vi "UHR-Fleezers Control (host) - 12.6.vi"() -> ()   [LabVIEW 2012] (continued)
                n2798 = xnode "Read/Write Control"("FPGA VI Reference In"=w3561, "error in"=w3560, "FPGA Trap Trig"=w3557) -> ("FPGA VI Reference Out"=w3559:T20, "error out"=w3558:errorcluster)
                n2799 = xnode "Read/Write Control"("FPGA VI Reference In"=w3559, "error in"=w3558, "TTrig?"=w3557) -> ()  [unwired: 2 out]
              }
            }
            n2800 = Select(t="Wait for trigger", s=w3544, f="Initialize") -> (s? t:f=w3552:string)
            n2801 = case shown="True" w3544 {
              tunnel: w3545 -> [_ w3564]
              tunnel: w3543 -> [_ w3573]
              tunnel: w3542 -> [_ w3572]
              frame False {
                n2802 = local write "Waiting"(FALSE ("Waiting")) -> ()
                "Initializing" <- TRUE ("Initializing")
              }
              frame True {
                n2803 = local read "Threshold (nm)"() -> (w3576:dbl)
                n2804 = local read "AOM X Cal (nm/MHz)"() -> (w3575:dbl)
                n2805 = Add(x=w3564, y=w3576) -> (x+y=w3577:dbl)
                n2806 = Divide(x=w3577, y=w3575) -> (x/y=w3574:dbl)
                n2807 = call "IR AOM freq to word.vi"("Frequency In (MHz)"=w3574) -> ("Frequency Word Out (double)"=w3571:dbl)
                n2808 = local write "Initializing"(FALSE ("Initializing")) -> ()
                n2809 = local write "Waiting"(TRUE ("Waiting")) -> ()
                n2810 = To Quad Integer(1:w3571) -> (0:w3570:i64)
                n2811 = xnode "Read/Write Control"("FPGA VI Reference In"=w3573, "error in"=w3572, "FPGA TTrig Thresh"=w3570) -> ("FPGA VI Reference Out"=w3567:T20, "error out"=w3566:errorcluster)
                n2812 = xnode "Read/Write Control"("FPGA VI Reference In"=w3567, "error in"=w3566, "FPGA Trap Trig"=TRUE) -> ()  [unwired: 2 out]
              }
            }
          }
        }
      }
    }
    n2813 = feedback-in #23(w3153) -> ()
    n2814 = feedback-in #24(w3150) -> ()
    n2815 = Split 1D Array(array=w3105, index=w3167) -> (first subarray=w3268:dbl[])  [unwired: 1 out]
    n2816 = feedback-in #25(w3268) -> ()
    n2817 = call-poly <vilib>:"Mean.vi"("X"=w3268) -> ("mean"=w3267:dbl)  [unwired: 1 out]
    "Bead Mean (nm)" <- w3267
    n2818 = Subtract(x=w3268, y=w3267) -> (x-y=w3266:dbl[])
    n2819 = Square(x=w3266) -> (x^2=w3265:dbl[])
    n2820 = call-poly <vilib>:"Mean.vi"("X"=w3265) -> ("mean"=w3264:dbl)  [unwired: 1 out]
    n2821 = Square Root(x=w3264) -> (sqrt(x)=w3263:dbl)
    n2822 = Multiply(x=10.0, y=w3263) -> (x*y=→"RMS (Ang)":dbl)
    n2823 = xnode ("Read/Write Control")("FPGA VI Reference In"=w3300, "error in"=w3299) -> ("FPGA VI Reference Out"=w3135:T20, "error out"=w3134:errorcluster, "AI2 Y Sum Set 1"=w3398:i16, "AI2 Y Sum Set 2"=w3397:i16, "AI1 X Set 1"=w3199:fxp<+/-,16,1>, "AI1 X Set 2"=w3198:fxp<+/-,16,1>, "Trap Pos FB Int Signal"=→"Trap Pos FB Int Signal":fxp<+/-,24,9>, "Trap Pos FB Int-Norm Signal"=→"Trap Pos FB Int-Norm Signal":fxp<+/-,16,1>, "Trap Pos FB Action"=w3192:i64, "Scanning"=→"AOD Scanning":bool, "Scan I"=→"AOD Scan I":u64, "Scanning MCL"=w3400:bool, "Scan I (MCL)"=→"MCL Scan I":u64, "Green FB Sum"=w3337:i16, "Trap Pos FB Action"=w3122:i64, "TTrig Fin Thresh"=w3118:i64, "Red FB Intensity"=w3099:i16, "Blue Intensity"=w3094:i16)
    "MCL Scanning" <- w3400
    "Trap Pos FB Action" <- w3192
    n2824 = Divide(x=w3099, y=3276.7) -> (x/y=w3098:dbl)
    "Red laser intensity (V)" <- w3098
    n2825 = Divide(x=w3094, y=3276.7) -> (x/y=w3093:dbl)
    "Blue laser intensity (V)" <- w3093
    n2826 = Divide(x=w3337, y=3276.7) -> (x/y=w3097:dbl)
    "Green laser intensity (V)" <- w3097
    n2827 = local read "FB Trig Integrate"() -> (w3116:u32)
    n2828 = Divide(x=w3122, y=w3116) -> (x/y=w3115:dbl)
    "TTrig Sig (Int)" <- w3115
    n2829 = Bundle(w3097, w3098, w3093) -> (→"Fluorescence laser intensities plot":cluster{dbl, dbl, dbl})  [unwired: 1 in]
    n2830 = Divide(x=w3118, y=w3116) -> (x/y=w3113:dbl)
    "TTrig Fin Thresh (Int)" <- w3113
    n2831 = local read "AOM X Cal (nm/MHz)"() -> (w3121:dbl)
    n2832 = local read "AI2 (V)"() -> (w3399:cluster{"Set 1":dbl, "Set 2":dbl})
    n2833 = Bundle By Name(cluster=w3399, "Set 1"=w3398, "Set 2"=w3397) -> (w3395:cluster{"Set 1":dbl, "Set 2":dbl})
    n2834 = Divide(x=w3192, y=327.67) -> (x/y=→"Action (%)":dbl)
    n2835 = local read "Trap X (AI1)"() -> (w3212:T10)
    n2836 = call "IR AOM word double to freq.vi"("Frequency Word In (double)"=w3113) -> ("Frequency Out (MHz)"=w3112:dbl)
    n2837 = call "IR AOM word double to freq.vi"("Frequency Word In (double)"=w3115) -> ("Frequency Out (MHz)"=w3114:dbl)
    n2838 = Divide(x=w3395, y=3276.7) -> (x/y=w3394:cluster{"Set 1":dbl, "Set 2":dbl})
    n2839 = Multiply(x=w3114, y=w3121) -> (x*y=w3120:dbl)
    "TTrig Sig (nm)" <- w3120
    n2840 = Multiply(x=w3112, y=w3121) -> (x*y=w3119:dbl)
    "TTrig Fin Thresh (nm)" <- w3119
    n2841 = local write "AI2 (V)"(w3394) -> ()
    n2842 = Bundle(cluster=w3212, "Trap 1"=w3199, "Trap 2"=w3198) -> (→"Trap X (AI1)":T10)
    n2843 = Bundle(w3120, w3119) -> (→"TTrig":cluster{dbl, dbl})  [unwired: 1 in]
    n2844 = flat-sequence "To save data" {
      tunnel: [w4484] -> w3418
      tunnel: [w4485] -> w3417
      tunnel: w3368 -> [w4478]
      tunnel: w3140 -> [w4482]
      tunnel: ["Save Calibration"] -> w3391
      tunnel: w3388 -> [w4481]
      tunnel: [w4474] -> w3387
      tunnel: [w4471] -> w3386
      tunnel: [w4468] -> w3385
      tunnel: w3367 -> [w4470]
      tunnel: w3282 -> [w4464]
      tunnel: [w4464] -> w3281
      tunnel: ["Start Saving"] -> w3251
      tunnel: [w4458] -> w3180
      tunnel: [w4457] -> w3179
      tunnel: w3418 -> [w4732]
      tunnel: w3417 -> [w4731]
      tunnel: w3181 -> [w4730]
      tunnel: w3391 -> [w4729]
      tunnel: w3387 -> [w4727]
      tunnel: w3386 -> [w4726]
      tunnel: w3385 -> [w4725]
      tunnel: w3260 -> [w4724]
      tunnel: w3292 -> [w4723]
      tunnel: w3281 -> [w4722]
      tunnel: w3251 -> [w4721]
      tunnel: w3249 -> [w4720]
      tunnel: w3077 -> [w4719]
      tunnel: w3180 -> [w4718]
      tunnel: w3179 -> [w4717]
      tunnel: w3178 -> [w4716]
      tunnel: w3101 -> [w4715]
      frame #0 {
        n2845 = Or(x="Save N Sets", y="Start Saving") -> (x .or. y?=w4465:bool)
        n2846 = To Double Precision Float(number=w4481) -> (double precision float=w4475:dbl)
        n2847 = Build Array(w4465, "Save Calibration", w4478, w4470) -> (w4480:bool[])
        n2848 = Compound Arithmetic op=OR("Save Calibration", w4478, w4465, w4470) -> (w4483:bool)
        n2849 = Boolean Array To Number(Boolean array=w4480) -> (number=w4477:u32)
        n2850 = feedback #27(FALSE ("Save APD Data\nwith Trap Data")) -> (w4459:bool)
        n2851 = feedback #28(refnum<k0> refnum) -> (w4486:refnum<file>)
        n2852 = feedback #29(refnum<k0> refnum) -> (w4461:refnum<file>)
        n2853 = feedback #30(FALSE ("Save APD Data\nwith Trap Data")) -> (w4469:bool)
        n2854 = feedback #31(refnum<k0> refnum) -> (w4472:refnum<file>)
        n2855 = feedback #32(0) -> (w4488:i32)
        n2856 = feedback #33() -> (w4476:u32)  [unwired: 1 out]
        n2857 = case shown="True" w4483 {
          tunnel: [w4495 1] -> w4484
          tunnel: w4488 -> [w4497 _]
          tunnel: [w4496 w4528] -> w4485
          tunnel: w4486 -> [w4496 _]
          tunnel: w4482 -> [_ w4546]
          tunnel: w4475 -> [_ w4544]
          tunnel: w4477 -> [_ w4547]
          tunnel: [w4494 w4527] -> w4474
          tunnel: w4476 -> [w4494 _]
          tunnel: [w4493 w4525] -> w4471
          tunnel: w4472 -> [w4493 _]
          tunnel: [w4492 w4524] -> w4468
          tunnel: w4469 -> [w4492 _]
          tunnel: "Start Saving" -> [_ w4522]
          tunnel: w4464 -> [_ w4521]
          tunnel: [w4491 w4513] -> w4457
          tunnel: w4461 -> [w4491 _]
          tunnel: [w4490 w4512] -> w4458
          tunnel: w4459 -> [w4490 _]
          frame False {
            n2858 = Increment(x=w4497) -> (x+1=w4495:i32)
          }
          frame True {
            w4518 = FALSE ("Start Saving")
            w4523 = 9.0  # File Version
            w4530 = FALSE ("prepend array or string size? (T)")
            w4529 = T28."big-endian, network order" ("byte order (0:big-endian, network order)")
            n2859 = local read "BD 1 Frequency 1 (MHz)"() -> (w4543:dbl)
            n2860 = local read "BD 2 Frequency 1 (MHz)"() -> (w4542:dbl)
            n2861 = local read "BD 1 Frequency 2 (MHz)"() -> (w4541:dbl)
            n2862 = local read "BD 2 Frequency 2 (MHz)"() -> (w4540:dbl)
            n2863 = local read "BD 1 Frequency 3 (MHz)"() -> (w4539:dbl)
            n2864 = local read "BD 2 Frequency 3 (MHz)"() -> (w4538:dbl)
            n2865 = Array Size(array=w4521) -> (size(s)=w4520:i32)
            n2866 = To Double Precision Float(number=w4520) -> (double precision float=w4519:dbl)
            n2867 = local write "Save Calibration"(w4518) -> ()
            n2868 = local write "Start Saving"(w4518) -> ()
            n2869 = Build Array("Save APD Data\nwith Trap Data", "Save Trap Pos. Data") -> (w4515:bool[])
            n2870 = Boolean Array To Number(Boolean array=w4515) -> (number=w4514:u32)
            n2871 = Build Array(w4543, w4542, w4541, w4540, w4539, w4538) -> (w4537:dbl[])
            n2872 = case shown="1, Default" w4547 {
              tunnel: w4546 -> [w4619 w4639 w4655 w4693]
              tunnel: w4519 -> [w4624 w4646 w4675 w4712]
              tunnel: w4544 -> [w4623 w4645 w4674 w4711]
              tunnel: [w4620 w4641 w4666 w4703] -> w4535
              tunnel: [w4611 "Cal sets to save" w4656 w4694] -> w4527
              tunnel: w4537 -> [w4621 w4642 w4668 w4705]
              tunnel: "Save APD Data\nwith Trap Data" -> [w4618 _ w4652 w4691]
              tunnel: [w4618 w4633 w4652 w4691] -> w4524
              tunnel: w4523 -> [w4614 w4634 w4650 w4689]
              tunnel: w4522 -> [w4613 _ _ _]
              tunnel: [w4604 w4633 w4649 w4679] -> w4512
              tunnel: "Save Trap Pos. Data" -> [w4604 _ w4649 w4679]
              tunnel: w4514 -> [w4603 _ w4648 w4678]
              frame 1, Default {
                # "timeseries"
                n2873 = case shown="True" "Profile" {
                  tunnel: [w4627 w4631] -> w4608
                  tunnel: [w4627 w4630] -> w4607
                  tunnel: [w4627 w4629] -> w4606
                  tunnel: [w4627 w4628] -> w4605
                  frame False {
                    w4627 = 0.0 ("f")
                  }
                  frame True {
                    n2874 = local read "Current Position"() -> (w4632:cluster{dbl, dbl, dbl})
                    n2875 = local read "Y change (mm)"() -> (w4628:dbl)
                    n2876 = Unbundle(w4632) -> (w4631:dbl, w4630:dbl, w4629:dbl)
                  }
                }
                n2877 = local read "Save ave N"() -> (w4626:dbl)
                n2878 = Multiply(x=w4626, y=w4619) -> (x*y=w4625:dbl)
                n2879 = To Double Precision Float(number=w4603) -> (double precision float=w4617:dbl)
                n2880 = Build Array(w4614, w4619, w4625, w4624, w4623, 0.0 ("f")) -> (w4622:dbl[])
                n2881 = Build Array(w4617, w4608, w4607, w4606, w4605) -> (w4615:dbl[])
                n2882 = Select(t=u32 4000000000, s=w4613, f="N sets to save") -> (s? t:f=w4611:u32)
                n2883 = Build Array (concatenate)(w4622, w4621, w4615) -> (w4620:dbl[])
              }
              frame 2 {
                w4636 = 0.0 ("f")
                w4633 = FALSE ("Save APD Data\nwith Trap Data")
                # "calibration"
                n2884 = Boolean To (0,1)(Boolean=w4633) -> (0, 1=w4638:i16)
                n2885 = To Double Precision Float(number=w4638) -> (double precision float=w4637:dbl)
                n2886 = Build Array(w4637, w4636, w4636, w4636, w4636) -> (w4635:dbl[])
                n2887 = Build Array(w4634, w4639, w4639, w4646, w4645, 1.0 ("t")) -> (w4643:dbl[])
                n2888 = Build Array (concatenate)(w4643, w4642, w4635) -> (w4641:dbl[])
                "Calibrating Trap..." <- TRUE ("Calibrating...")
              }
              frame 4 {
                w4653 = 0.0 ("f")
                # "scan dir (x/y = 0/1)"
                # "cycles/step"
                # "n scans (f/b)"
                # "steps"
                # "freq. range"
                # "AOD raster scan"
                n2889 = local read "Number of F/B Scans (AOD)"() -> (w4660:u16)
                n2890 = local read "Cycles/step (AOD)"() -> (w4662:u64)
                n2891 = local read "Scan Range (MHz)"() -> (w4665:dbl)
                n2892 = local read "Scan steps (AOD)"() -> (w4664:u64)
                n2893 = local read "Scan BD"() -> (w4672:bool)
                n2894 = local read "Save ave N"() -> (w4677:dbl)
                n2895 = Boolean To (0,1)(Boolean=w4672) -> (0, 1=w4671:i16)
                n2896 = To Double Precision Float(number=w4660) -> (double precision float=w4659:dbl)
                n2897 = To Double Precision Float(number=w4664) -> (double precision float=w4663:dbl)
                n2898 = To Double Precision Float(number=w4662) -> (double precision float=w4661:dbl)
                n2899 = To Double Precision Float(number=w4671) -> (double precision float=w4670:dbl)
                n2900 = Multiply(x=w4677, y=w4655) -> (x*y=w4676:dbl)
                n2901 = To Double Precision Float(number=w4648) -> (double precision float=w4654:dbl)
                n2902 = Build Array(w4654, w4653, w4653, w4653, w4653) -> (w4651:dbl[])
                n2903 = local read "N sets should be saved"() -> (w4657:dbl)
                n2904 = Build Array(w4670, w4665, w4663, w4661, w4659) -> (w4667:dbl[])
                n2905 = Build Array(w4650, w4655, w4676, w4675, w4674, 2.0 ("t")) -> (w4669:dbl[])
                n2906 = Round Toward +Infinity(x=w4657) -> (ceil(x): smallest int >= x=w4658:dbl)
                n2907 = Build Array (concatenate)(w4669, w4668, w4651, w4667) -> (w4666:dbl[])
                n2908 = To Unsigned Long Integer(number=w4658) -> (unsigned 32bit integer=w4656:u32)
              }
              frame 8 {
                w4686 = 0.0 ("f")
                # "MCL raster scan"
                n2909 = local read "Number of scans (MCL)"() -> (w4681:u64)
                n2910 = local read "Scan lines (y)"() -> (w4680:u64)
                n2911 = local read "2D or 1D Scan"() -> (w4683:bool)
                n2912 = local read "Scan Range (V)\n(of steps)"() -> (w4702:dbl)
                n2913 = local read "Fast Scan Dir"() -> (w4709:bool)
                n2914 = local read "Cycles/step (MCL)"() -> (w4699:u64)
                n2915 = local read "Scan steps (MCL)"() -> (w4701:u64)
                n2916 = Select(t=w4680, s=w4683, f=w4681) -> (s? t:f=w4682:u64)
                n2917 = Boolean To (0,1)(Boolean=w4683) -> (0, 1=w4685:i16)
                n2918 = local read "Save ave N"() -> (w4714:dbl)
                n2919 = local read "Initial X"() -> (w4688:dbl)
                n2920 = local read "Initial Y"() -> (w4687:dbl)
                n2921 = To Double Precision Float(number=w4685) -> (double precision float=w4684:dbl)
                n2922 = Boolean To (0,1)(Boolean=w4709) -> (0, 1=w4708:i16)
                n2923 = To Double Precision Float(number=w4682) -> (double precision float=w4697:dbl)
                n2924 = To Double Precision Float(number=w4701) -> (double precision float=w4700:dbl)
                n2925 = To Double Precision Float(number=w4699) -> (double precision float=w4698:dbl)
                n2926 = To Double Precision Float(number=w4708) -> (double precision float=w4707:dbl)
                n2927 = Multiply(x=w4714, y=w4693) -> (x*y=w4713:dbl)
                n2928 = To Double Precision Float(number=w4678) -> (double precision float=w4692:dbl)
                n2929 = local read "N sets should be saved (MCL)"() -> (w4695:dbl)
                n2930 = Build Array(w4692, w4684, w4686, w4686, w4686) -> (w4690:dbl[])
                n2931 = Build Array(w4707, w4702, w4700, w4698, w4697, w4688, w4687) -> (w4704:dbl[])
                n2932 = Build Array(w4689, w4693, w4713, w4712, w4711, 3.0 ("t")) -> (w4706:dbl[])
                n2933 = Round Toward +Infinity(x=w4695) -> (ceil(x): smallest int >= x=w4696:dbl)
                n2934 = Build Array (concatenate)(w4706, w4705, w4690, w4704) -> (w4703:dbl[])
                n2935 = To Unsigned Long Integer(number=w4696) -> (unsigned 32bit integer=w4694:u32)
              }
            }
            n2936 = local read "Index"() -> (w4552:dbl)
            n2937 = call "Create new save file.vi"("Insert"="", "Ext"=".dat", "Index In"=w4552) -> ("Path Out"=w4508:path, "Index Out"=w4526:dbl)
            n2938 = local write "Save file name"(w4508) -> ()
            n2939 = local write "Index"(w4526) -> ()
            n2940 = local write "Save index"(w4526) -> ()
            n2941 = Array Size(array=w4535) -> (size(s)=w4536:i32)
            n2942 = Open/Create/Replace File(file path (use dialog)=w4508, operation (0:open)=T29."create", access (0:read/write)=enum16{"read/write", "read-only", "write-only"}."write-only") -> (refnum out=w4549:refnum<file>)  [unwired: 1 in, 4 out]
            n2943 = local write "Saving..."(TRUE ("Saving...")) -> ()
            n2944 = To Double Precision Float(number=w4536) -> (double precision float=w4534:dbl)
            n2945 = String Length(string="Comment (data description)") -> (length=w4533:i32)
            n2946 = To Double Precision Float(number=w4533) -> (double precision float=w4532:dbl)
            n2947 = Deny Access(7:w4549) -> (3:w4548:refnum<file>)  [unwired: 1 in, 2 out]
            n2948 = Build Array (concatenate)(w4534, w4535, w4532) -> (w4507:dbl[])
            n2949 = case "If fluorescence data to be saved" shown="True" w4524 {
              tunnel: w4508 -> [_ w4602]
              tunnel: [refnum<k0> refnum w4582] -> w4525
              frame False {
              }
              frame True {
                w4581 = 0.0
                n2950 = local read "APD Integration Time (s)"() -> (w4587:dbl)
                n2951 = local read "N APD Samp/step"() -> (w4580:dbl)
                n2952 = local read "Number of APDs"() -> (w4579:u8)
                n2953 = Path To String(path=w4602) -> (string=w4601:string)
                n2954 = String Length(string=w4601) -> (length=w4600:i32)
                n2955 = Subtract(x=w4600, y=4) -> (x-y=w4598:i32)
                n2956 = String Subset(string=w4601, length (rest)=w4598) -> (substring=w4597:string)  [unwired: 1 out]
                n2957 = Build Array(w4587, w4580, w4579, w4581, w4581, w4581, w4581, w4581) -> (w4584:dbl[])
                n2958 = Concatenate Strings(w4597, "_fl.dat" ("string")) -> (w4595:string)
                n2959 = Array Size(array=w4584) -> (size(s)=w4586:i32)
                n2960 = String To Path(string=w4595) -> (path=w4591:path)
                n2961 = Open/Create/Replace File(file path (use dialog)=w4591, operation (0:open)=T29."create", access (0:read/write)=enum16{"read/write", "read-only", "write-only"}."write-only") -> (refnum out=w4592:refnum<file>)  [unwired: 1 in, 4 out]
                n2962 = Deny Access(7:w4592) -> (3:w4588:refnum<file>)  [unwired: 1 in, 2 out]
                n2963 = To Double Precision Float(number=w4586) -> (double precision float=w4585:dbl)
                n2964 = Build Array (concatenate)(w4585, w4584) -> (w4583:dbl[])
                n2965 = Write to Binary File(file (use dialog)=w4588, data=w4583, 5:FALSE ("prepend array or string size? (T)"), 9:T28."big-endian, network order" ("byte order (0:big-endian, network order)")) -> (refnum out=w4582:refnum<file>)  [unwired: 1 in, 3 out]
              }
            }
            n2966 = case shown="True" w4512 {
              tunnel: w4508 -> [_ w4563]
              tunnel: [refnum<k0> refnum w4562] -> w4513
              frame False {
              }
              frame True {
                w4558 = 0.0 ("element")
                n2967 = Path To String(path=w4563) -> (string=w4577:string)
                n2968 = Build Array(w4558, w4558, w4558, w4558, w4558, w4558, w4558, w4558) -> (w4559:dbl[])
                n2969 = String Length(string=w4577) -> (length=w4576:i32)
                n2970 = Subtract(x=w4576, y=4) -> (x-y=w4574:i32)
                n2971 = Array Size(array=w4559) -> (size(s)=w4561:i32)
                n2972 = String Subset(string=w4577, length (rest)=w4574) -> (substring=w4573:string)  [unwired: 1 out]
                n2973 = To Double Precision Float(number=w4561) -> (double precision float=w4560:dbl)
                n2974 = Concatenate Strings(w4573, "_pos.dat" ("string")) -> (w4571:string)
                n2975 = Build Array (concatenate)(w4560, w4559) -> (w4557:dbl[])
                n2976 = String To Path(string=w4571) -> (path=w4567:path)
                n2977 = Open/Create/Replace File(file path (use dialog)=w4567, operation (0:open)=T29."create", access (0:read/write)=enum16{"read/write", "read-only", "write-only"}."write-only") -> (refnum out=w4568:refnum<file>)  [unwired: 1 in, 4 out]
                n2978 = Deny Access(7:w4568) -> (3:w4564:refnum<file>)  [unwired: 1 in, 2 out]
                n2979 = Write to Binary File(file (use dialog)=w4564, data=w4557, 5:FALSE ("prepend array or string size? (T)"), 9:T28."big-endian, network order" ("byte order (0:big-endian, network order)")) -> (refnum out=w4562:refnum<file>)  [unwired: 1 in, 3 out]
              }
            }
            n2980 = Write to Binary File(file (use dialog)=w4548, data=w4507, 5:w4530, 9:w4529) -> (refnum out=w4531:refnum<file>)  [unwired: 1 in, 3 out]
            n2981 = Write to Binary File(file (use dialog)=w4531, data="Comment (data description)", 5:w4530, 9:w4529) -> (refnum out=w4528:refnum<file>)  [unwired: 1 in, 3 out]
            n2982 = local read "connection reference"() -> (w4510:T17)
            n2983 = Bundle("Comment (data description)"="Comment (data description)", "Channel 1 Buffer"="Channel 1 Buffer", "Channel 2 Buffer"="Channel 2 Buffer", "Channel 3 Buffer"="Channel 3 Buffer", "Title"="Title", "DNA Construct"="DNA Construct", "Bead diameter"="Bead diameter", "Name"="Name") -> (w4498:T47)  [unwired: 1 in]
            n2984 = call "MattFileCreator-v9.vi"("Comments"=w4498, "Input Array"=w4507, "File path"=w4508, "table"="labview", "connection reference"=w4510) -> ("connection reference out"=w4509:T17)  [unwired: 5 in, 1 out]
            n2985 = local write "connection reference"(w4509) -> ()
          }
        }
        n2986 = feedback-in #27(w4458) -> ()
        n2987 = feedback-in #28(w4485) -> ()
        n2988 = feedback-in #29(w4457) -> ()
        n2989 = feedback-in #30(w4468) -> ()
        n2990 = feedback-in #31(w4471) -> ()
        n2991 = feedback-in #32(w4484) -> ()
        n2992 = feedback-in #33(w4474) -> ()
      }
      frame #1 {
        n2993 = local read "Saving..."() -> (w4728:bool)
        n2994 = case shown="True" w4728 {
          tunnel: w4732 -> [_ w4743]
          tunnel: w4731 -> [_ w4757]
          tunnel: w4730 -> [_ w4753]
          tunnel: w4729 -> [_ w4752]
          tunnel: w4727 -> [_ w4751]
          tunnel: w4726 -> [_ w4746]
          tunnel: w4725 -> [_ w4745]
          tunnel: w4724 -> [_ w4744]
          tunnel: w4723 -> [_ w4742]
          tunnel: w4722 -> [_ w4740]
          tunnel: w4721 -> [_ w4739]
          tunnel: w4720 -> [_ w4738]
          tunnel: w4719 -> [_ w4737]
          tunnel: w4718 -> [_ w4736]
          tunnel: w4717 -> [_ w4735]
          tunnel: w4716 -> [_ w4734]
          tunnel: w4715 -> [_ w4733]
          frame False {
          }
          frame True {
            n2995 = Multiply(x=w4743, y=w4742) -> (x*y=→"Time (s)":dbl)
            n2996 = Less Or Equal?(x=w4743, y=w4751) -> (x <= y?=w4755:bool)
            n2997 = Or(x="Stop Saving", y="Abort save 2") -> (x .or. y?=w4747:bool)
            n2998 = Not(x=w4747) -> (.not. x?=w4756:bool)
            n2999 = And(x=w4755, y=w4756) -> (x .and. y?=w4754:bool)
            n3000 = case shown="True" w4754 {
              tunnel: w4757 -> [w4764 w4855]
              tunnel: [0.0 w4858] -> w4750
              tunnel: w4743 -> [_ w4856]
              tunnel: w4751 -> [_ w4857]
              tunnel: w4753 -> [_ w4852]
              tunnel: w4752 -> [_ _]
              tunnel: w4746 -> [w4762 w4845]
              tunnel: w4745 -> [w4761 w4846]
              tunnel: w4744 -> [_ w4844]
              tunnel: w4740 -> [_ w4843]
              tunnel: w4739 -> [_ w4767]
              tunnel: w4738 -> [_ w4836]
              tunnel: w4737 -> [_ w4783]
              tunnel: w4736 -> [w4758 w4800]
              tunnel: w4735 -> [w4759 w4799]
              tunnel: w4734 -> [_ w4796]
              tunnel: w4733 -> [_ w4794]
              frame False {
                w4760 = FALSE
                n3001 = Close File(refnum=w4764) -> ()  [unwired: 1 in, 2 out]
                n3002 = case shown="True" w4761 {
                  tunnel: w4762 -> [_ w4766]
                  frame False {
                  }
                  frame True {
                    n3003 = Close File(refnum=w4766) -> ()  [unwired: 1 in, 2 out]
                  }
                }
                n3004 = case shown="True" w4758 {
                  tunnel: w4759 -> [_ w4765]
                  frame False {
                  }
                  frame True {
                    n3005 = Close File(refnum=w4765) -> ()  [unwired: 1 in, 2 out]
                  }
                }
                n3006 = local write "Raster Scanning..."(w4760) -> ()
                n3007 = local write "Calibrating Trap..."(w4760) -> ()
                n3008 = call <vilib>:"Beep.vi"() -> ()  [unwired: 3 in, 9 out]
                n3009 = local write "Stop Saving"(w4760) -> ()
                "Saving..." <- w4760
              }
              frame True {
                n3010 = local read "Calibrating Trap..."() -> (w4847:bool)
                n3011 = case "Write fl. data" shown="True" w4846 {
                  tunnel: w4845 -> [_ w4881]
                  tunnel: w4844 -> [_ w4880]
                  frame False {
                  }
                  frame True {
                    n3012 = Write to Binary File(file (use dialog)=w4881, data=w4880, 5:FALSE ("prepend array or string size? (T)"), 9:T28."big-endian, network order" ("byte order (0:big-endian, network order)")) -> ()  [unwired: 1 in, 4 out]
                  }
                }
                n3013 = Greater?(x="Save ave N", y=1.0) -> (0:w4850:bool)
                n3014 = Not(x=w4847) -> (.not. x?=w4849:bool)
                n3015 = And(x=w4849, y=w4850) -> (x .and. y?=w4797:bool)
                n3016 = case shown="True" w4797 {
                  tunnel: w4796 -> [w4861 w4872]
                  tunnel: [w4861 w4864] -> w4795
                  tunnel: "Save ave N" -> [_ w4865]
                  frame False {
                  }
                  frame True {
                    w4862 = 2 ("dimension size")
                    n3017 = Array Size(array=w4872) -> (size(s)=w4866:i32)
                    n3018 = Divide(x=w4866, y=w4862) -> (x/y=w4870:dbl)
                    n3019 = Reshape Array(w4872, w4870, w4862) -> (w4871:u64[][])
                    n3020 = Transpose 2D Array(2D array=w4871) -> (transposed array=w4869:u64[][])
                    n3021 = for {
                      tunnel: w4869 -> [w4874] mode=indexing
                      tunnel: [w4873] -> w4863 mode=indexing
                      tunnel: w4865 -> [w4875]
                      workers-P: _ -> [_]
                      n3022 = call "downsample 1D array - U64.vi"("Ave N"=w4875, "Array In"=w4874) -> ("Array Out"=w4873:u64[])  [unwired: 1 in]
                    }
                    n3023 = Transpose 2D Array(2D array=w4863) -> (transposed array=w4868:u64[][])
                    n3024 = Divide(x=w4866, y=w4865) -> (x/y=w4867:dbl)
                    n3025 = Reshape Array(w4868, w4867) -> (w4864:u64[])
                  }
                }
                n3026 = case shown="True" w4797 {
                  tunnel: w4852 -> [w4884 w4896]
                  tunnel: [w4884 w4888] -> w4848
                  tunnel: "Save ave N" -> [_ w4889]
                  tunnel: w4843 -> [_ w4887]
                  frame False {
                  }
                  frame True {
                    n3027 = Array Size(array=w4896) -> (size(s)=w4890:i32)
                    n3028 = Array Size(array=w4887) -> (size(s)=w4886:i32)
                    n3029 = Divide(x=w4890, y=w4886) -> (x/y=w4894:dbl)
                    n3030 = Reshape Array(w4896, w4894, w4886) -> (w4895:i16[][])
                    n3031 = Transpose 2D Array(2D array=w4895) -> (transposed array=w4893:i16[][])
                    n3032 = for {
                      tunnel: w4893 -> [w4899] mode=indexing
                      tunnel: [w4898] -> w4885 mode=indexing
                      tunnel: w4889 -> [w4897]
                      workers-P: _ -> [_]
                      n3033 = call "downsample 1D array - I16.vi"("Ave N"=w4897, "Array In"=w4899) -> ("Array Out"=w4898:i16[])  [unwired: 1 out]
                    }
                    n3034 = Transpose 2D Array(2D array=w4885) -> (transposed array=w4892:i16[][])
                    n3035 = Divide(x=w4890, y=w4889) -> (x/y=w4891:dbl)
                    n3036 = Reshape Array(w4892, w4891) -> (w4888:i16[])
                  }
                }
                n3037 = Index Array(array=w4783, index=2) -> (element=w4784:waveform(dbl))
                n3038 = Index Array(array=w4783, index=1) -> (element=w4817:waveform(dbl))
                n3039 = Index Array(array=w4783, index=0) -> (element=w4819:waveform(dbl))
                n3040 = Unbundle By Name(w4784) -> ("Y"=w4786:dbl[])
                n3041 = Unbundle By Name(w4817) -> ("Y"=w4821:dbl[])
                n3042 = Unbundle By Name(w4819) -> ("Y"=w4829:dbl[])
                n3043 = case "Write trap pos. data" shown="True" w4800 {
                  tunnel: w4799 -> [_ w4877]
                  tunnel: w4795 -> [_ w4876]
                  frame False {
                  }
                  frame True {
                    n3044 = Write to Binary File(file (use dialog)=w4877, data=w4876, 5:FALSE ("prepend array or string size? (T)"), 9:T28."big-endian, network order" ("byte order (0:big-endian, network order)")) -> ()  [unwired: 1 in, 4 out]
                  }
                }
                n3045 = Write to Binary File(file (use dialog)=w4855, data=w4848, 5:FALSE ("prepend array or string size? (T)"), 9:T28."big-endian, network order" ("byte order (0:big-endian, network order)")) -> ()  [unwired: 1 in, 4 out]
                n3046 = feedback #34(w4786) -> (w4787:dbl[])
                n3047 = Build Array (concatenate)(w4787, w4786) -> (w4782:dbl[])
                n3048 = Select(t=w4786, s=w4767, f=w4782) -> (s? t:f=w4772:dbl[])
                n3049 = feedback-in #34(w4772) -> ()
                n3050 = feedback #35(w4821) -> (w4823:dbl[])
                n3051 = Build Array (concatenate)(w4823, w4821) -> (w4822:dbl[])
                n3052 = Select(t=w4821, s=w4767, f=w4822) -> (s? t:f=w4811:dbl[])
                n3053 = feedback-in #35(w4811) -> ()
                n3054 = feedback #36(w4829) -> (w4842:dbl[])
                n3055 = Build Array (concatenate)(w4842, w4829) -> (w4841:dbl[])
                n3056 = Select(t=w4829, s=w4767, f=w4841) -> (s? t:f=w4816:dbl[])
                n3057 = feedback-in #36(w4816) -> ()
                n3058 = Divide(x=w4856, y=w4857) -> (x/y=w4859:dbl)
                n3059 = Multiply(x=w4859, y=100.0) -> (x*y=w4858:dbl)
                n3060 = Build Array(w4816, w4811, w4772) -> (→"Saved APD":dbl[][])
                n3061 = Array Size(array=w4816) -> (size(s)=w4834:i32)
                n3062 = Unbundle By Name(w4836) -> ("Y"=w4840:dbl[])
                n3063 = Subtract(x=w4834, y="N pts to average") -> (x-y=w4769:i32)
                n3064 = Multiply(x="N pts to average", y=u16 2) -> (x*y=w4812:u16)
                n3065 = Subtract(x=w4834, y=w4812) -> (x-y=w4770:i32)
                n3066 = feedback #37(w4840) -> (w4839:dbl[])
                n3067 = Build Array (concatenate)(w4839, w4840) -> (w4838:dbl[])
                n3068 = Select(t=w4840, s=w4767, f=w4838) -> (s? t:f=w4837:dbl[])
                "Trap Delta Graph" <- w4837
                n3069 = feedback-in #37(w4837) -> ()
                n3070 = Array Subset(array=w4816, index=w4769, length="N pts to average") -> (w4833:dbl[])
                n3071 = Array Subset(array=w4816, index=w4770, length="N pts to average") -> (w4832:dbl[])
                n3072 = Array Subset(array=w4811, index=w4769, length="N pts to average") -> (w4814:dbl[])
                n3073 = Array Subset(array=w4811, index=w4770, length="N pts to average") -> (w4813:dbl[])
                n3074 = Array Subset(array=w4772, index=w4769, length="N pts to average") -> (w4781:dbl[])
                n3075 = Array Subset(array=w4772, index=w4770, length="N pts to average") -> (w4780:dbl[])
                n3076 = Index Array(array=w4794, index=0) -> (element=w4792:waveform(dbl))
                n3077 = call-poly <vilib>:"Mean.vi"("X"=w4833) -> ("mean"=w4831:dbl)  [unwired: 1 out]
                n3078 = call-poly <vilib>:"Mean.vi"("X"=w4814) -> ("mean"=w4810:dbl)  [unwired: 1 out]
                n3079 = call-poly <vilib>:"Mean.vi"("X"=w4832) -> ("mean"=w4830:dbl)  [unwired: 1 out]
                n3080 = call-poly <vilib>:"Mean.vi"("X"=w4813) -> ("mean"=w4809:dbl)  [unwired: 1 out]
                n3081 = call-poly <vilib>:"Mean.vi"("X"=w4781) -> ("mean"=w4779:dbl)  [unwired: 1 out]
                n3082 = call-poly <vilib>:"Mean.vi"("X"=w4780) -> ("mean"=w4778:dbl)  [unwired: 1 out]
                n3083 = Unbundle By Name(w4792) -> ("Y"=w4790:dbl[])
                n3084 = Subtract(x=w4810, y=w4809) -> (x-y=w4801:dbl)
                "Delta Fl. 2" <- w4801
                n3085 = Subtract(x=w4779, y=w4778) -> (x-y=w4773:dbl)
                "Delta Fl. 3" <- w4773
                n3086 = Subtract(x=w4831, y=w4830) -> (x-y=w4828:dbl)
                "Delta Fl. 1" <- w4828
                n3087 = feedback #38(w4790) -> (w4789:dbl[])
                n3088 = Build Array (concatenate)(w4789, w4790) -> (w4791:dbl[])
                n3089 = Initialize Array(w4828, 1 ("dimension size")) -> (w4825:dbl[])
                n3090 = Initialize Array(w4801, 1 ("dimension size")) -> (w4806:dbl[])
                n3091 = Initialize Array(w4773, 1 ("dimension size")) -> (w4775:dbl[])
                n3092 = Select(t=w4790, s=w4767, f=w4791) -> (s? t:f=w4788:dbl[])
                "Saved trap pos" <- w4788
                n3093 = feedback-in #38(w4788) -> ()
                n3094 = feedback #39(w4825) -> (w4826:dbl[])
                n3095 = Build Array (concatenate)(w4826, w4825) -> (w4824:dbl[])
                n3096 = feedback #40(w4806) -> (w4807:dbl[])
                n3097 = feedback #41(w4775) -> (w4776:dbl[])
                n3098 = Build Array (concatenate)(w4807, w4806) -> (w4805:dbl[])
                n3099 = Build Array (concatenate)(w4776, w4775) -> (w4774:dbl[])
                n3100 = Select(t=w4825, s=w4767, f=w4824) -> (s? t:f=w4804:dbl[])
                n3101 = feedback-in #39(w4804) -> ()
                n3102 = Select(t=w4806, s=w4767, f=w4805) -> (s? t:f=w4803:dbl[])
                n3103 = feedback-in #40(w4803) -> ()
                n3104 = Select(t=w4775, s=w4767, f=w4774) -> (s? t:f=w4768:dbl[])
                n3105 = feedback-in #41(w4768) -> ()
                n3106 = Build Array(w4804, w4803, w4768) -> (→"Save APD Deriv":dbl[][])
              }
            }
            "Progress" <- w4750
            "Progress 2" <- w4750
          }
        }
      }
    }
    n3107 = local read "wait to reset values"() -> (w3402:bool)
    n3108 = Not(x=w3400) -> (.not. x?=w3403:bool)
    n3109 = And(x=w3403, y=w3402) -> (x .and. y?=w3404:bool)
    n3110 = case "Part of MCL raster scanning: returns to initial positions after scan done" shown="True" w3404 {
      tunnel: w3135 -> [w4278 w4285]
      tunnel: [w4278 w4284] -> w3406
      tunnel: w3134 -> [w4277 w4283]
      tunnel: [w4277 w4282] -> w3401
      frame False {
      }
      frame True {
        w4293 = 10.0 ("y")
        w4292 = 32767.0 ("y")
        # "to return scan values\nafter a synchronous \nAOM scan"
        n3111 = local read "AO2"() -> (w4286:dbl)
        n3112 = local read "AO1"() -> (w4287:dbl)
        n3113 = local write "wait to reset values"(FALSE ("wait to reset values")) -> ()
        n3114 = Multiply(x=w4287, y=w4292) -> (x*y=w4289:dbl)
        n3115 = Multiply(x=w4286, y=w4292) -> (x*y=w4291:dbl)
        n3116 = Divide(x=w4289, y=w4293) -> (x/y=w4288:dbl)
        n3117 = Divide(x=w4291, y=w4293) -> (x/y=w4290:dbl)
        n3118 = To Word Integer(number=w4288) -> (16bit integer=w4294:i16)
        n3119 = To Word Integer(number=w4290) -> (16bit integer=w4295:i16)
        n3120 = local read "Total Counts (ticks)"() -> (w4279:u16)
        n3121 = xnode "Read/Write Control"("FPGA VI Reference In"=w4285, "error in"=w4283, "AO1"=w4294, "AO2"=w4295, "MCL count"=w4279) -> ("FPGA VI Reference Out"=w4284:T20, "error out"=w4282:errorcluster)
        n3122 = local read "Scan Range (V)\n(of steps)"() -> (w4280:dbl)
        n3123 = property on="Scan Range (V)\n(of steps)" class="DigNum (strict)"("Val(Sgnl)"=w4280) -> ()  [unwired: 2 in, 2 out]
      }
    }
    n3124 = node-c288() -> ()  [unwired: 2 out]
  }
  n3125 = flat-sequence "Video" {
    tunnel: [w4909] -> w114
    tunnel: w114 -> [w4949]
    frame #0 {
      n3126 = while {
        stop <- w4901 continue-if-true
        n3127 = call "Close Video Capture.vi"() -> ("error code OUT"=w4903:i32)
        n3128 = Equal?(x=w4903, y=0) -> (x = y?=w4901:bool)
      }
      n3129 = local write "Stop All"(FALSE ("Stop All")) -> ()
    }
    frame #1 {
      n3130 = call "DMR_Init.vi"() -> ()  [unwired: 3 out]
    }
    frame #2 {
      w4904 = "DE245428202"  # MSU fleezers card #
      (unwired) "DE019116701"  # Illinois fleezers card #
      # "Setting the destination format to Mono8 makes sure that the image can be displayed in the intensity plot."
      n3131 = call "DMR_GetDevice.vi"("search string IN"=w4904) -> ("device handle OUT"=w4927:i32)  [unwired: 4 in, 2 out]
      n3132 = call "DMR_OpenDevice.vi"("device handle IN"=w4927) -> ("driver handle OUT"=w4910:i32)  [unwired: 4 out]
      n3133 = call "DMR_FindList.vi"("flags IN"=u32 0 ("flags"), "list name IN"="" ("String"), "list type IN"=T48."camera descriptions", "driver handle IN"=w4910) -> ("list handle OUT"=w4913:i32)  [unwired: 2 out]
      n3134 = call "DMR_FindList.vi"("flags IN"=u32 0 ("flags"), "list name IN"="Base", "list type IN"=T48."setting", "driver handle IN"=w4910) -> ("list handle OUT"=w4911:i32)  [unwired: 2 out]
      n3135 = call "OBJ_GetHandle.vi"("object name IN"="VideoStandard", "list handle IN"=w4913) -> ("object handle OUT"=w4907:i32)  [unwired: 3 out]
      n3136 = call "OBJ_GetHandle.vi"("object name IN"="PixelFormat", "list handle IN"=w4911) -> ("object handle OUT"=w4921:i32)  [unwired: 3 out]
      n3137 = call "OBJ_SetS.vi"("value index IN"=0, "value IN"="NTSC M", "object handle IN"=w4907) -> ()  [unwired: 2 out]
      n3138 = call "OBJ_SetS.vi"("value index IN"=0, "value IN"="Mono8" ("value"), "object handle IN"=w4921) -> ()  [unwired: 2 out]
      n3139 = call "OBJ_GetHandle.vi"("object name IN"="VideoChannel", "list handle IN"=w4911) -> ("object handle OUT"=w4917:i32)  [unwired: 3 out]
      n3140 = while {
        tunnel: [w4931] -> w4909
        tunnel: w4910 -> [w4928]
        stop <- w4929 continue-if-true
        n3141 = call "DMR_ImageRequestSingle.vi"("request control IN"=0, "driver handle IN"=w4928) -> ("error code OUT"=w4930:i32, "driver handle OUT"=w4931:i32)  [unwired: 2 out]
        n3142 = Equal To 0?(x=w4930) -> (x = 0?=w4929:bool)
      }
      n3143 = call "OBJ_SetI.vi"("value index IN"=0, "value IN"=3 ("Video channel"), "object handle IN"=w4917) -> ()  [unwired: 2 out]
    }
    frame #3 {
      w4937 = T18 0 items=["Grayscale (U8)", "Grayscale (I16)", "Grayscale (SGL)", "Complex (CSG)", "RGB (U32)", "HSL (U32)", "RGB (U64)"] ("Image Type")
      w4945 = T18 0 items=["Grayscale (U8)", "Grayscale (I16)", "Grayscale (SGL)", "Complex (CSG)", "RGB (U32)", "HSL (U32)", "RGB (U64)"] ("Image Type")
      n3144 = for "Create Greyscale map" {
        N: 256 -> [_]
        tunnel: [w4951] -> w4934 mode=indexing
        workers-P: _ -> [_]
        i -> [w4954]
        n3145 = To Unsigned Byte Integer(number=w4954) -> (unsigned 8bit integer=w4950:u8)
        n3146 = Join Numbers(hi=w4950, lo=w4950) -> ((hi.lo)=w4953:u16)
        n3147 = Join Numbers(hi=w4950, lo=w4950) -> ((hi.lo)=w4952:u16)
        n3148 = Join Numbers(hi=w4953, lo=w4952) -> ((hi.lo)=w4951:u32)
      }
      n3149 = call "IMAQ Create"("Image Name"="Scaled video", "Image Type"=w4937) -> ("New Image"=w4936:T2)  [unwired: 2 in, 2 out]
      n3150 = call "IMAQ Create"("Image Name"="Main video", "Image Type"=w4945) -> ("New Image"=w4946:T2)  [unwired: 2 in, 2 out]
      n3151 = node-c288(0 ("Processor")) -> (w4944:T23)  [unwired: 3 out]
      n3152 = Initialize Array(u32 0 ("Window Number (0...15)"), 480 ("dimension size"), 640 ("dimension size")) -> (w4939:u32[][])
      n3153 = timed-loop {
        tunnel: w4949 -> [w4971]
        tunnel: [w4970] -> w4948
        tunnel: w4946 -> [w4969]
        timing: w4944 -> [_]
        timing-out: [_] -> w4943
        tunnel: w4939 -> [w4958]
        tunnel: w4936 -> [w4956]
        tunnel: w4934 -> [w4955]
        stop <- w4957 stop-if-true
        # "This block performs the \nactual image capture."
        n3154 = node-c288() -> ()  [unwired: 2 out]
        n3155 = local read "Stop All"() -> (w4957:bool)
        n3156 = Reciprocal(x="Video Capture Rate (Hz)") -> (1/x=w4961:dbl)
        n3157 = Multiply(x=w4961, y=1000.0) -> (x*y=w4959:dbl)
        n3158 = call "DMR_ImageRequestWaitFor.vi"("queue number IN"=0, "timeout(ms) IN"=500, "driver handle IN"=w4971) -> ("error code OUT"=w4975:i32, "request number OUT"=w4972:i32, "driver handle OUT"=w4973:i32)
        n3159 = feedback #42(T49 refnum ("Avi Refnum")) -> (w4963:T49)
        n3160 = case shown="True" "New Video File" {
          tunnel: [T49 refnum ("Avi Refnum") w4992] -> w4965
          tunnel: [FALSE TRUE] -> w4966
          tunnel: w4963 -> [_ w4988]
          frame False {
          }
          frame True {
            n3161 = call "Create new save file.vi"("Ext"=".avi" ("string"), "Index In"="Video Index") -> ("Path Out"=w4984:path, "Index Out"=w4985:dbl)  [unwired: 1 in]
            "Path Out" <- w4984
            n3162 = Not Equal?(x=w4988, y=T49 refnum ("Avi Refnum")) -> (x != y?=w4989:bool)
            n3163 = Increment(x=w4985) -> (x+1=w4994:dbl)
            n3164 = case shown="True" w4989 {
              tunnel: w4988 -> [_ w4995]
              frame False {
              }
              frame True {
                n3165 = call "IMAQ AVI Close"("Avi Refnum"=w4995) -> ()  [unwired: 1 in, 10 out]
              }
            }
            n3166 = local write "Video Index"(w4994) -> ()
            n3167 = call "IMAQ AVI Create"("Frames Per Second"=u32 30, "AVI Path"=w4984) -> ("Avi Refnum"=w4992:T49)  [unwired: 5 in, 4 out]
          }
        }
        n3168 = Equal To 0?(x=w4975) -> (x = 0?=w4974:bool)
        n3169 = Select(t=w4965, s=w4966, f=w4963) -> (s? t:f=w4964:T49)
        n3170 = feedback-in #42(w4964) -> ()
        n3171 = case shown="True" w4974 {
          tunnel: w4973 -> [w4996 w5030]
          tunnel: w4972 -> [_ w5029]
          tunnel: [w4996 w5026] -> w4970
          tunnel: w4969 -> [_ w5011]
          tunnel: w4958 -> [_ w5015]
          tunnel: w4964 -> [_ w5013]
          tunnel: w4956 -> [_ w5008]
          tunnel: w4955 -> [_ w5007]
          frame False {
          }
          frame True {
            w5020 = u32 0 ("X-offset IN")
            n3172 = call "DMR_GetImageRequestBufferData.vi"("driver handle IN"=w5030, "request number IN"=w5029) -> ("width OUT"=w5019:i32, "height OUT"=w5018:i32, "driver handle OUT"=w5025:i32, "request number OUT"=w5024:i32, "bytes per pixel OUT"=w5021:i32)  [unwired: 13 out]
            n3173 = call "DMR_GetImageRequestBufferImageData.vi"("driver handle IN"=w5025, "request number IN"=w5024, "bytes per pixel IN"=w5021, "X-offset IN"=w5020, "Y-offset IN"=w5020, "height IN"=w5018, "width IN"=w5019) -> ("driver handle OUT"=w5023:u32, "request number OUT"=w5022:u32, "image OUT"=w5000:u32[][])  [unwired: 10 out]
            n3174 = Transpose 2D Array(2D array=w5000) -> (transposed array=w5006:u32[][])
            n3175 = Select(t=w5006, s="Flip Y (or X)", f=w5000) -> (s? t:f=w5005:u32[][])
            n3176 = call "DMR_ImageRequestUnlock.vi"("request number IN"=w5022, "driver handle IN"=w5023) -> ("driver handle OUT"=w5028:i32)  [unwired: 1 in, 2 out]
            n3177 = for {
              tunnel: w5005 -> [w5065] mode=indexing
              tunnel: [w5064] -> w5003 mode=indexing
              n3178 = Reverse 1D Array(array=w5065) -> (reversed array=w5064:u32[])
            }
            n3179 = call "DMR_ImageRequestSingle.vi"("request control IN"=0, "driver handle IN"=w5028) -> ("driver handle OUT"=w5026:i32)  [unwired: 3 out]
            n3180 = Transpose 2D Array(2D array=w5003) -> (transposed array=w5004:u32[][])
            n3181 = Select(t=w5004, s="Flip Y (or X)", f=w5003) -> (s? t:f=w5001:u32[][])
            n3182 = Select(t=w5001, s="Flip Image", f=w5000) -> (s? t:f=w4998:u32[][])
            n3183 = case shown="True" "Averaging" {
              tunnel: w4998 -> [w5068 w5073]
              tunnel: [w5068 w5072] -> w5012
              tunnel: w5015 -> [_ w5070]
              frame False {
              }
              frame True {
                (unwired) 1
                w5078 = 1
                n3184 = feedback #43(w5070) -> (w5069:u32[][])
                n3185 = Add(x=w5073, y=w5069) -> (x+y=w5074:u32[][])
                n3186 = Select(t=w5070, s="Reset Averaging", f=w5074) -> (s? t:f=w5076:u32[][])
                n3187 = feedback-in #43(w5076) -> ()
                n3188 = feedback #44(w5078) -> (w5071:i32)
                n3189 = Divide(x=w5074, y=w5071) -> (x/y=w5075:dbl[][])
                n3190 = Increment(x=w5071) -> (x+1=w5079:i32)
                n3191 = To Unsigned Long Integer(number=w5075) -> (unsigned 32bit integer=w5072:u32[][])
                n3192 = Select(t=w5078, s="Reset Averaging", f=w5079) -> (s? t:f=w5077:i32)
                n3193 = feedback-in #44(w5077) -> ()
              }
            }
            n3194 = case shown="True" "Zoom video window" {
              tunnel: w5012 -> [_ w5044]
              tunnel: w5008 -> [_ w5043]
              frame False {
              }
              frame True {
                n3195 = To Double Precision Float(number=w5044) -> (double precision float=w5041:dbl[][])
                n3196 = In Range and Coerce(upper limit="Intensity Upper", x=w5041, lower limit="Intensity Lower") -> (coerced(x)=w5040:dbl[][])  [unwired: 1 out]
                n3197 = Subtract(x="Intensity Upper", y="Intensity Lower") -> (x-y=w5037:dbl)
                n3198 = Subtract(x=w5040, y="Intensity Lower") -> (x-y=w5038:dbl[][])
                n3199 = Divide(x=w5038, y=w5037) -> (x/y=w5039:dbl[][])
                n3200 = Multiply(x=255.0, y=w5039) -> (x*y=w5035:dbl[][])
                n3201 = To Unsigned Byte Integer(number=w5035) -> (unsigned 8bit integer=w5042:u8[][])
                n3202 = call "IMAQ ArrayToImage"("Image Pixels (U8)"=w5042, "Image"=w5043) -> ("Image Out"=w5031:T2)  [unwired: 4 in, 5 out]
                n3203 = First Call?() -> (First Call?: T/F=w5032:bool)
                n3204 = case shown="True" w5032 {
                  tunnel: w5031 -> [w5045 w5056]
                  frame False {
                    n3205 = flat-sequence {
                      tunnel: w5045 -> [w5051]
                      frame #0 {
                        w5048 = FALSE ("Get/Set Status? (Set)")
                        w5047 = 0 ("Window Number (0...15)")
                        n3206 = call "IMAQ WindSize"("Get/Set Status? (Set)"=w5048, "Window Number"=w5047) -> ("Width & Height out"=→"Window Size":cluster{"Width":i32, "Height":i32})  [unwired: 4 in, 2 out]
                        n3207 = call "IMAQ WindMove"("Window Number (0...15)"=w5047, "Get/Set Status? (Set)"=w5048) -> ("Coordinates (screen)"=→"Window Position":cluster{"X Position":i32, "Y Position":i32})  [unwired: 3 in, 1 out]
                        n3208 = call "IMAQ WindDraw"("Resize to Image Size? (Y)"=FALSE, "Window Number (0...15)"=w5047, "Image"=w5051) -> ()  [unwired: 7 in, 2 out]
                      }
                      frame #1 {
                        n3209 = call "IMAQ WindZoom 2"("Center Point"="Center Point", "Zoom to Fit? (False)"=FALSE, "Zoom Factor"="Zoom Factor") -> ()  [unwired: 5 in, 4 out]
                      }
                    }
                  }
                  frame True {
                    n3210 = flat-sequence {
                      tunnel: w5056 -> [w5059]
                      tunnel: [w5057] -> w5055
                      tunnel: w5055 -> [w5061]
                      frame #0 {
                        w5058 = TRUE ("Resize to Image Size? (Y)")
                        w5057 = 0 ("Window Number (0...15)")
                        n3211 = call "IMAQ WindNonTearing"("Window Number"=w5057, "NonTearing? (True)"=w5058) -> ()  [unwired: 8 in, 2 out]
                        n3212 = call "IMAQ WindDraw"("Resize to Image Size? (Y)"=w5058, "Window Number (0...15)"=w5057, "Image"=w5059) -> ()  [unwired: 7 in, 2 out]
                      }
                      frame #1 {
                        n3213 = call "IMAQ WindSize"("Scrollbars? (N)"=FALSE, "Width & Height"="Initial Window Size", "Window Number"=w5061) -> ()  [unwired: 3 in, 3 out]
                        n3214 = call "IMAQ WindMove"("Window Number (0...15)"=w5061, "Coordinates (screen)"="Initial Window Position") -> ()  [unwired: 3 in, 2 out]
                      }
                    }
                  }
                }
              }
            }
            n3215 = To Unsigned Byte Integer(number=w5012) -> (unsigned 8bit integer=w5010:u8[][])
            n3216 = call "IMAQ ArrayToImage"("Image Pixels (U8)"=w5010, "Image"=w5011) -> ("Image Out"=w5009:T2)  [unwired: 4 in, 5 out]
            "Primary Video Display" <- w5009
            n3217 = case shown="True" "Save Video" {
              tunnel: w5013 -> [_ w5067]
              tunnel: w5009 -> [_ w5066]
              frame False {
              }
              frame True {
                n3218 = call "IMAQ AVI Write Frame"("Image"=w5066, "Avi Refnum"=w5067) -> ()  [unwired: 2 in, 8 out]
              }
            }
            n3219 = case shown="True" "Save Image" {
              tunnel: w5010 -> [_ w5082]
              tunnel: w5007 -> [_ w5081]
              frame False {
              }
              frame True {
                n3220 = call <vilib>:"Flatten Pixmap.vi"("colors"=w5081, "8-bit pixmap"=w5082) -> ("image data"=w5088:T50)  [unwired: 4 in, 5 out]
                n3221 = call "Create new save file.vi"("Insert"="video_frame_" ("string"), "Ext"=".bmp" ("string"), "Index In"="Image Index") -> ("Path Out"=w5084:path, "Index Out"=w5089:dbl)
                n3222 = Increment(x=w5089) -> (x+1=w5083:dbl)
                n3223 = local write "Image Index"(w5083) -> ()
                n3224 = call <vilib>:"Write BMP File.vi"("image data"=w5088, "path to BMP file"=w5084) -> ()  [unwired: 1 in, 9 out]
              }
            }
          }
        }
        n3225 = node-c288(w4959) -> ()  [unwired: 1 out]
      }
      n3226 = node-c288(w4943) -> ()  [unwired: 1 out]
      n3227 = call "DMR_CloseDevice.vi"("driver handle IN"=w4948) -> ()  [unwired: 1 in, 4 out]
    }
    frame #4 {
      n3228 = call "DMR_Close.vi"() -> ()  [unwired: 1 out]
    }
  }
  n3229 = timed-loop "Rough control of MCL mirror stage (debugging)" {
    tunnel: w16 -> [w5096]
    tunnel: [w5095] -> w254
    timing: w10 -> [_]
    timing-out: [_] -> w9
    stop <- w5095 stop-if-true
    n3230 = node-c288() -> ()  [unwired: 2 out]
    n3231 = case shown="1" "MCL Mode" {
      tunnel: w5096 -> [_ w5099 w5146]
      frame 0, Default {
      }
      frame 1 {
        n3232 = node-c288() -> (w5101:T23)  [unwired: 4 out]
        n3233 = timed-loop "Oscillate MCL mirror" {
          timing: w5101 -> [_]
          timing-out: [_] -> w5100
          tunnel: w5099 -> [w5140]
          i -> [w5139]
          stop <- w5102 stop-if-true
          n3234 = node-c288() -> (w5138:i64)  [unwired: 1 out]
          n3235 = Multiply(x="AO1", y=32767.0) -> (x*y=w5134:dbl)
          n3236 = Multiply(x="AO2", y=32767.0) -> (x*y=w5129:dbl)
          n3237 = Divide(x=w5134, y=10.0) -> (x/y=w5135:dbl)
